vi "process safe state.vi"(8 "error in":errorcluster, 9 "result allocation":T1, 10 "parameters":T1, 11 "ActiveFrontEndModule runtime in":refnum<class "ActiveFrontEndModule runtime.lvclass">) -> (0 "error out":errorcluster, 1 "results":T1, 2 "parameter allocation":T1, 3 "ActiveFrontEndModule runtime out":refnum<class "ActiveFrontEndModule runtime.lvclass">)   [LabVIEW 2017, in "ActiveFrontEndModule runtime.lvclass"]
doc: "Provides an interface for information processing by a module when in a safe state. This interface simply calls the normal processing function. However, if child modules need to have custom logic during safe-state operation, this can be implemented here.\nNI Tag Bus Module Framework 1.0.2.34\nNI Systems Engineering"
uses:
  ActiveFrontEndModule runtime.lvclass
  <vilib>/NI/Tag Bus/table/data table.ctl
  result user data.ctl
  ActiveFrontEndModule runtime.lvclass/ActiveFrontEndModule runtime.ctl
  <vilib>/NI/Tag Bus/table/data table.lvlib
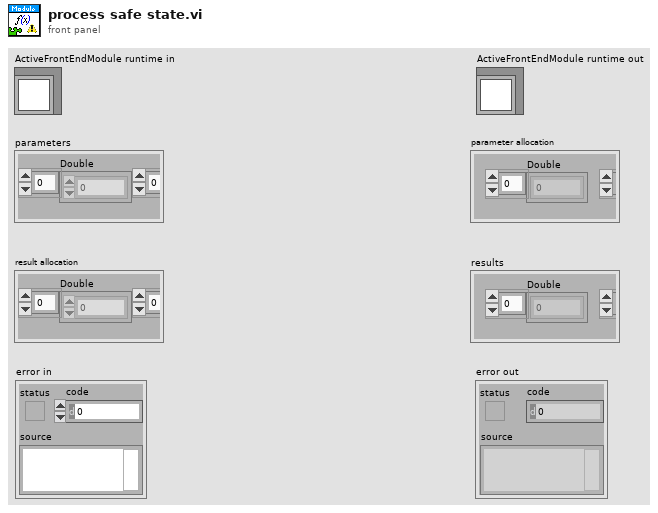
[diagram p1: front panel]
types:
  T1 = typedef "tag bus.lvlib/data table.lvlib/data table.ctl" = cluster{"Double":dbl[], "Single":sgl[], "I64":i64[], "I32":i32[], "I16":i16[], "I8":i8[], "U64":u64[], "U32":u32[], "U16":u16[], "U8":u8[], "Boolean":bool[], "String":string[], "Array of Double":cluster{"DBL Array":dbl[]}[], "Array of Single":cluster{"SGL Array":sgl[]}[], "Array of I64":cluster{"I64 Array":i64[]}[], "Array of I32":cluster{"I32 Array":i32[]}[], "Array of I16":cluster{"I16 Array":i16[]}[], "Array of I8":cluster{"I8 Array":i8[]}[], "Array of U64":cluster{"U64 Array":u64[]}[], "Array of U32":cluster{"U32 Array":u32[]}[], "Array of U16":cluster{"U16 Array":u16[]}[], "Array of U8":cluster{"U8 Array":u8[]}[], "Array of Boolean":cluster{"Boolean Array":bool[]}[], "Array of String":cluster{"String Array":string[]}[]}
  T2 = typedef "ActiveFrontEndModule runtime.lvclass/result user data.ctl" = cluster{"fmwk_placeholder":i32}
  T3 = typedef "ActiveFrontEndModule configuration.lvclass/result data indices.ctl" = cluster{"fmwk_placeholder":i32}
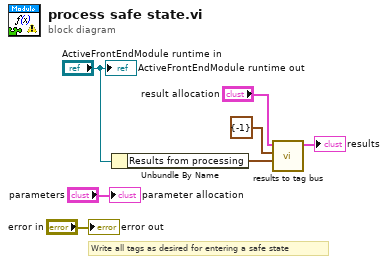
[diagram p0: block diagram]
diagram:
  # "Write all tags as desired for entering a safe state"
  n1 = Unbundle By Name("ActiveFrontEndModule runtime in") -> ("Results from processing"=w5:T3)
  n2 = call "results to tag bus.vi"("indices"=w5, "data cluster"=T2 {"fmwk_placeholder"=-1}, "tag bus in"="result allocation") -> ("tag bus out"=→"results":T1)  [unwired: 8 in]
  "ActiveFrontEndModule runtime out" <- "ActiveFrontEndModule runtime in"
  "error out" <- "error in"
  "parameter allocation" <- "parameters"
